vi "BCD Decode Integer.vi"(11 "BCD encoded value":bool[](array[boolean])) -> (3 "integer":i64)   [LabVIEW 2020, in "Encoding and Decoding.lvlib"]
uses:
  Encoding and Decoding/Encoding and Decoding.lvlib
  9a65bfc0-0d77-4ef3-ab58-63df1e1caa90.vi
panel:
  in  "base":u8(ring)=10 items=["Binary (2)"=2, "Octal (8)"=8, "Decimal (10)"=10, "Hexadecimal (16)"=16]
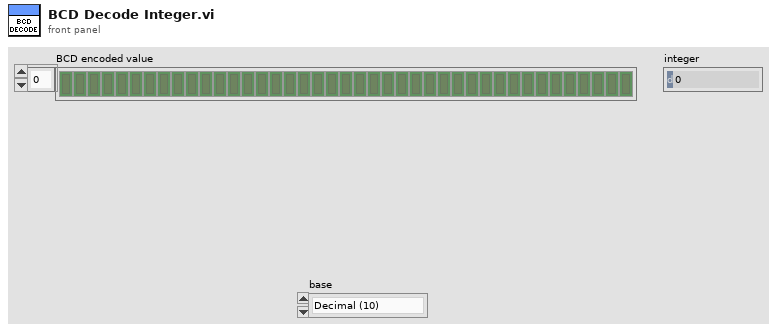
[diagram p1: front panel]
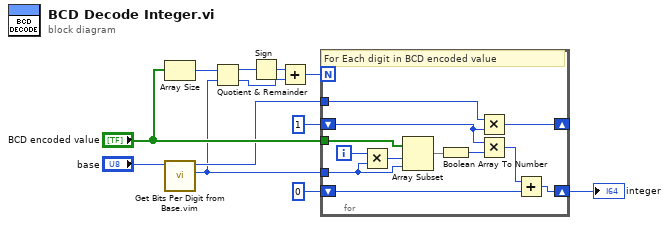
[diagram p0: block diagram]
diagram:
  n1 = Array Size(array="BCD encoded value") -> (size(s)=w9:i32)
  n2 = call "Get Bits Per Digit from Base.vim"("base"="base") -> ("bits per digit"=w1:i32, "base"=w2:i32)  [unwired: 9 in]
  n3 = Quotient & Remainder(x=w9, y=w1) -> (x-y*floor(x/y)=w12:i32, floor(x/y)=w11:i32)
  n4 = Sign(1:w12) -> (0:w10:i32)
  n5 = Add(x=w10, y=w11) -> (x+y=w5:i32)
  n6 = for {
    N: w5 -> [_]
    tunnel: w1 -> [w13]
    shift-right: [w19] -> w6
    shift-left: i64 0 ("x") -> [w18]
    tunnel: "BCD encoded value" -> [w24]
    shift-right: [w15] -> _
    shift-left: i64 1 ("x") -> [w14]
    tunnel: w2 -> [w16]
    i -> [w23]
    # "For Each digit in BCD encoded value"
    n7 = Multiply(x=w23, y=w13) -> (x*y=w22:i32)
    n8 = Array Subset(array=w24, index=w22, length=w13) -> (w21:bool[])
    n9 = Boolean Array To Number(Boolean array=w21) -> (number=w20:u32)
    n10 = Multiply(x=w16, y=w14) -> (x*y=w15:i64)
    n11 = Multiply(x=w14, y=w20) -> (x*y=w17:i64)
    n12 = Add(x=w17, y=w18) -> (x+y=w19:i64)
  }
  "integer" <- w6
